vi "Labview Server.vi"() -> ()   [LabVIEW 2019]
panel:
  in  "stop":bool
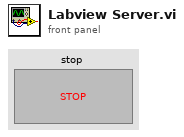
[diagram p1: front panel]
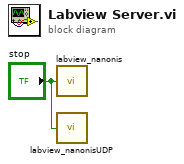
[diagram p0: block diagram]
diagram:
  n1 = call "labview_nanonis.vi"("stop"="stop") -> ()
  n2 = call "labview_nanonisUDP.vi"("stop"="stop") -> ()
